vi "DualTrigs.vi"() -> ()   [LabVIEW 2022 SP3]
uses:
  <vilib>/Utility/error.llb/DialogType.ctl
  <vilib>/DAQmx/create/channels.llb/DAQmx Create Channel (CO-Pulse Generation-Time).vi
  <vilib>/DAQmx/configure/timing.llb/DAQmx Timing (Implicit).vi
  <vilib>/DAQmx/configure/trigger.llb/DAQmx Start Trigger (Digital Edge).vi
  <resource>/objmgr/daqmx.rc
panel:
  in  "Stop":bool caption="stop"
  in  "Counter(s) 2":tag="Dev1/ctr2" caption="Counter(s)"
  in  "Initial Delay":sgl format="%#_6e"
  in  "Idle State 2":i32(ring)=10214 caption="Idle State" items=["High"=10192, "Low"=10214]
  in  "Trigger Edge 2":i32(ring)=10280 caption="Trigger Edge" items=["Rising"=10280, "Falling"=10171]
  in  "Low Ticks":sgl=3e-05 format="%#_6e"
  in  "High Ticks":sgl=0.0005 format="%#_6e"
  in  "Trigger Source":tag="/Dev1/Ctr1Gate"
  in  "Trigger Edge":i32(ring)=10280 items=["Rising"=10280, "Falling"=10171]
  in  "Source":tag="/Dev1/PFI34" caption="Trigger Source"
  in  "Initial delay":dbl format="%.2e"
  in  "Low Time":dbl=2e-05 format="%.2e"
  in  "High Time":dbl=2e-05 format="%.2e"
  in  "Idle State":i32(ring)=10214 items=["High"=10192, "Low"=10214]
  in  "Counter(s)":tag="Dev1/ctr1"
  # "Phase Level Gate"
  # "Twin Trigs"
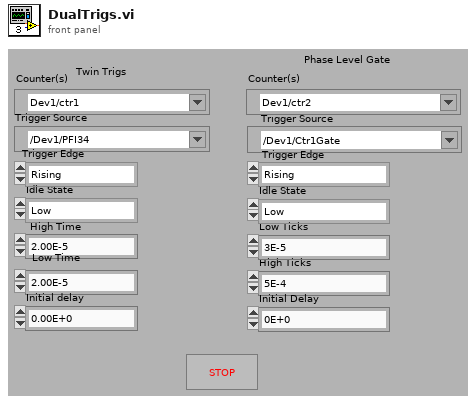
[diagram p1: front panel]
types:
  T1 = typedef "DialogType.ctl" = u16
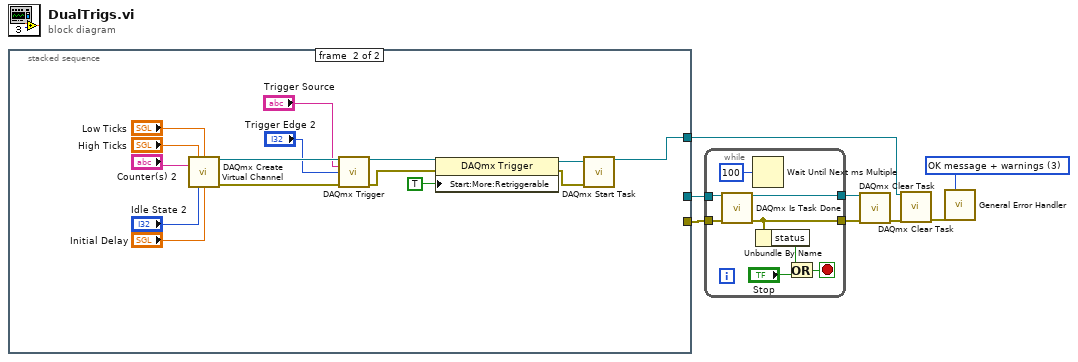
[diagram p0: block diagram]
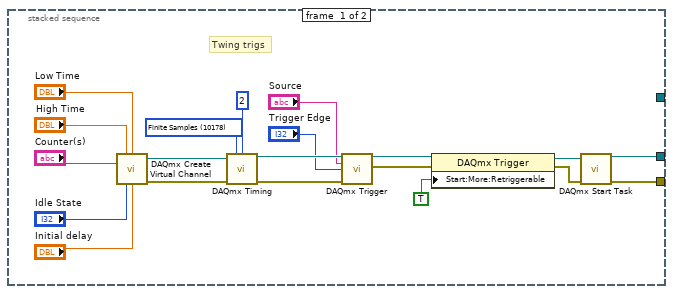
[diagram p2: hidden frame]
diagram:
  w8 = T1 3 items=["no dialog", "OK message", "continue or stop message", "OK message + warnings", "continue/stop + warnings"] ("type of dialog (OK msg:1)")
  n1 = stacked-sequence {
    tunnel: [w10 _] -> w7
    tunnel: [w9 _] -> w6
    tunnel: [_ w43] -> w1
    frame #0 {
      w26 = 10178 items=["Finite Samples"=10178, "Continuous Samples"=10123] ("sample mode")
      # "Twing trigs"
      n2 = call-poly <vilib>:"DAQmx Create Virtual Channel.vi"("high time"="High Time", "low time"="Low Time", "counter"="Counter(s)", "idle state"="Idle State", "initial delay"="Initial delay") -> ("task out"=w27:refnum<k21>, "error out"=w28:errorcluster)  [unwired: 4 in, 5 out]
      n3 = call-poly <vilib>:"DAQmx Timing.vi"("task/channels in"=w27, "sample mode"=w26, "samples per channel"=2, "error in"=w28) -> ("task out"=w20:refnum<k21>, "error out"=w19:errorcluster)  [unwired: 10 out]
      n4 = call-poly <vilib>:"DAQmx Trigger.vi"("task/channels in"=w20, "source"="Source", "edge"="Trigger Edge", "error in"=w19) -> ("task out"=w15:refnum<k21>, "error out"=w14:errorcluster)  [unwired: 10 out]
      n5 = property class="DAQmx Trigger"(reference=w15, error in=w14, "Start:More:Retriggerable"=TRUE) -> (reference out=w13:refnum<k21>, error out=w12:errorcluster)
      n6 = call <vilib>:"DAQmx Start Task.vi"("task/channels in"=w13, "error in"=w12) -> ("task out"=w10:refnum<k21>, "error out"=w9:errorcluster)  [unwired: 12 out]
    }
    frame #1 {
      n7 = call-poly <vilib>:"DAQmx Create Virtual Channel.vi"("high time"="High Ticks", "low time"="Low Ticks", "counter"="Counter(s) 2", "idle state"="Idle State 2", "initial delay"="Initial Delay") -> ("task out"=w40:refnum<k21>, "error out"=w39:errorcluster)  [unwired: 4 in, 5 out]
      n8 = call-poly <vilib>:"DAQmx Trigger.vi"("task/channels in"=w40, "source"="Trigger Source", "edge"="Trigger Edge 2", "error in"=w39) -> ("task out"=w32:refnum<k21>, "error out"=w31:errorcluster)  [unwired: 10 out]
      n9 = property class="DAQmx Trigger"(reference=w32, error in=w31, "Start:More:Retriggerable"=TRUE) -> (reference out=w30:refnum<k21>, error out=w29:errorcluster)
      n10 = call <vilib>:"DAQmx Start Task.vi"("task/channels in"=w30, "error in"=w29) -> ("task out"=w43:refnum<k21>)  [unwired: 13 out]
    }
  }
  n11 = while {
    tunnel: [w44] -> w5
    tunnel: [w45] -> w4
    tunnel: w7 -> [w47]
    tunnel: w6 -> [w46]
    stop <- w49 stop-if-true
    n12 = call <vilib>:"DAQmx Is Task Done.vi"("task/channels in"=w47, "error in"=w46) -> ("task out"=w44:refnum<k21>, "error out"=w45:errorcluster)  [unwired: 12 out]
    n13 = Wait Until Next ms Multiple(millisecond multiple=u32 100) -> ()  [unwired: 1 out]
    n14 = Unbundle By Name(w45) -> ("status"=w50:bool)
    n15 = Or(x=w50, y="Stop") -> (x .or. y?=w49:bool)
  }
  n16 = call <vilib>:"DAQmx Clear Task.vi"("task in"=w5, "error in"=w4) -> ("error out"=w3:errorcluster)  [unwired: 13 out]
  n17 = call <vilib>:"DAQmx Clear Task.vi"("task in"=w1, "error in"=w3) -> ("error out"=w2:errorcluster)  [unwired: 13 out]
  n18 = call <vilib>:"General Error Handler.vi"("type of dialog (OK msg:1)"=w8, "error in (no error)"=w2) -> ()  [unwired: 1 in, 13 out]
